vi "MTS_SaveImagePng.vi"(5 "Save .png":bool=TRUE, 6 "Tree Refnum":refnum<vi>, 7 ".pt3 File Name":path, 8 "error in":errorcluster, 11 "Image":i32[][](array[numeric])) -> (0 "error out":errorcluster)   [LabVIEW 8.6]
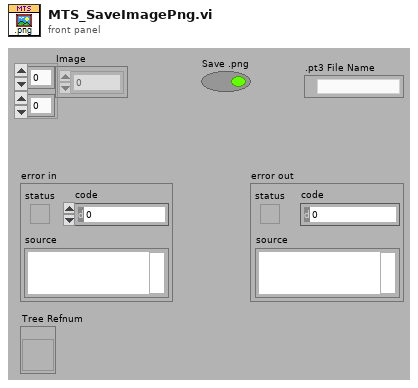
[diagram p1: front panel]
types:
  T1 = enum16{"unknown", "pt3 File", "png Image", "bmp Image"}
  T2 = enum16{"not a pt3 File", "Image File", "Point Measurement", "Auto Point"}
  T3 = typedef "Image Type" = u32
  T4 = typedef "IMAQ Image.ctl" = refnum<image>
  T5 = cluster{"File No":i32, "File Path":path, "Parent File":i32, "File Type":enum16{"unknown", "pt3 File", "png Image", "bmp Image"}, "Measurement Type":enum16{"not a pt3 File", "Image File", "Point Measurement", "Auto Point"}, "Upper Left":cluster{"x-Position":dbl, "y-Position":dbl, "z-Position":dbl}, "Pixels":i32[], "Picture Size":dbl[], "Scan Axis":enum32{"x-y", "x-z", "y-z"}}
  T6 = cluster{"x-Position":dbl, "y-Position":dbl, "z-Position":dbl}
  T7 = cluster{"Picture Size":dbl[], "Pixels":i32[], "Upper Left":cluster{"x-Position":dbl, "y-Position":dbl, "z-Position":dbl}}
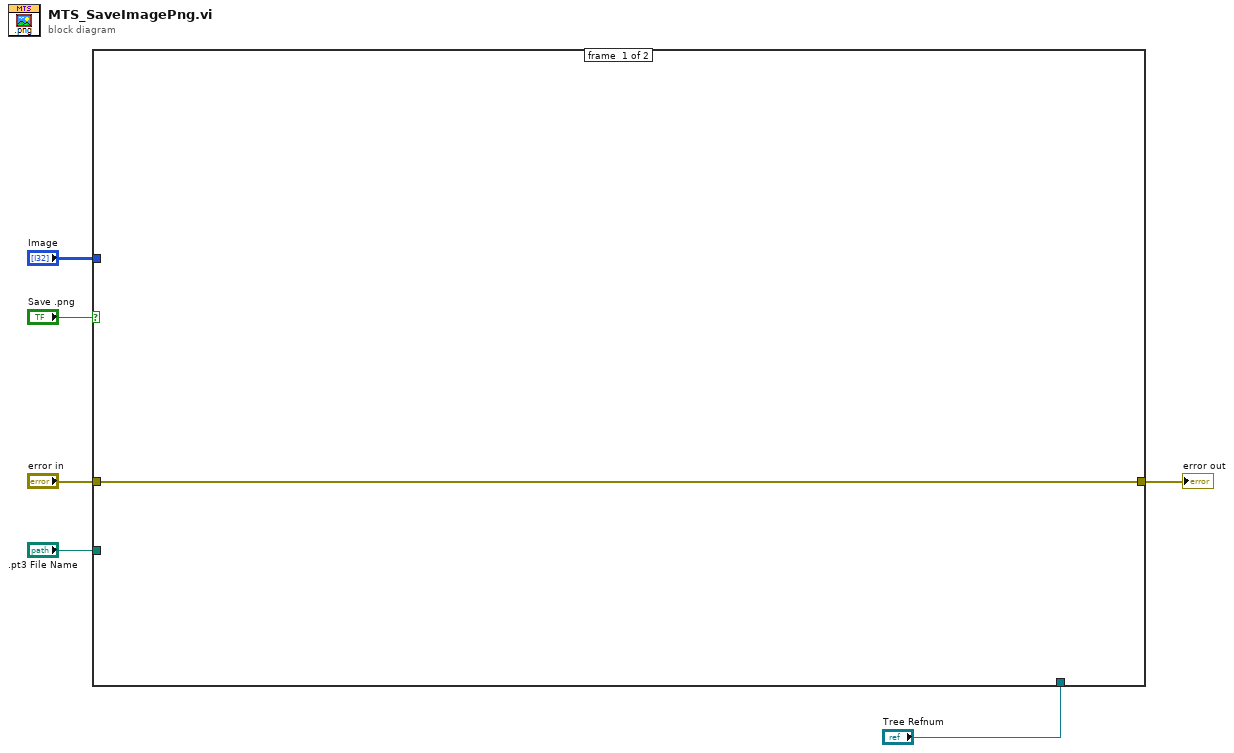
[diagram p0: block diagram]
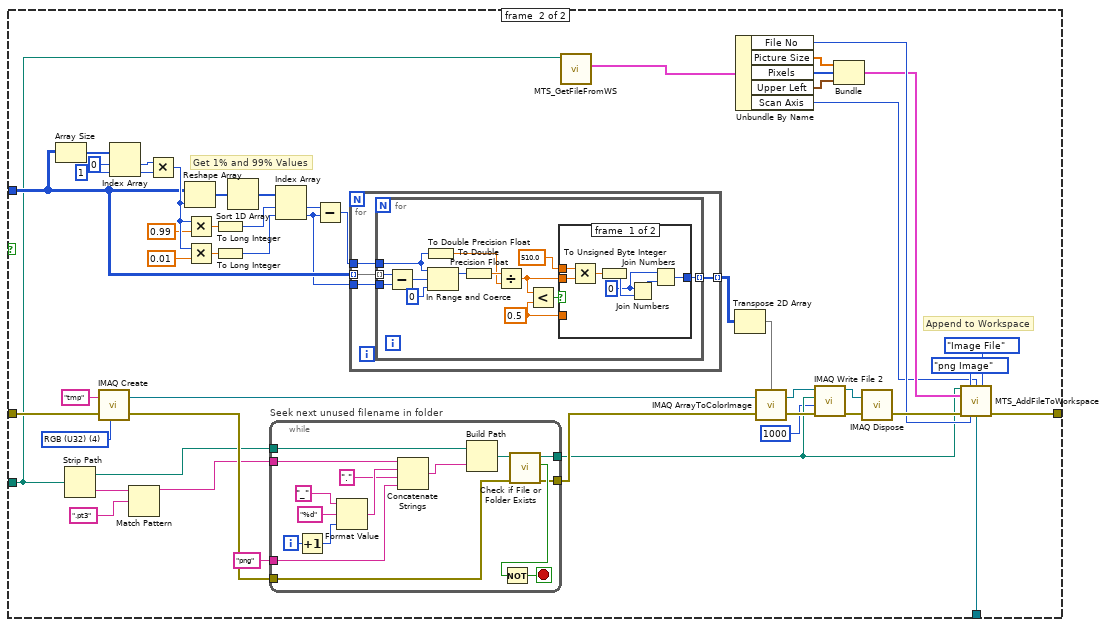
[diagram p2: hidden frame]
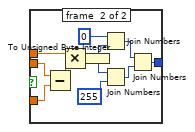
[diagram p3: hidden frame]
diagram:
  n1 = case shown="True" "Save .png" {
    tunnel: "Image" -> [_ w40]
    tunnel: "error in" -> [w7 w43]
    tunnel: [w7 w23] -> w3
    tunnel: ".pt3 File Name" -> [_ w9]
    tunnel: "Tree Refnum" -> [_ w22]
    frame #0 {
    }
    frame #1 {
      w41 = T3 4 items=["Grayscale (U8)", "Grayscale (I16)", "Grayscale (SGL)", "Complex (CSG)", "RGB (U32)", "HSL (U32)", "RGB (U64)", "Grayscale (U16)"] ("Image Type")
      # "Append to Workspace"
      # "Get 1% and 99% Values"
      n2 = Array Size(array=w40) -> (size(s)=w57:i32[])
      n3 = Strip Path(path=w9) -> (stripped path=w27:path, name=w31:string)
      n4 = call "IMAQ Create"("Image Name"="tmp", "Image Type"=w41, "error in (no error)"=w43) -> ("New Image"=w36:T4, "error out"=w29:errorcluster)  [unwired: 2 in]
      n5 = Index Array(array=w57, index #1=0 ("index"), index #2=1 ("index")) -> (element #1=w54:i32, element #2=w53:i32)
      n6 = Match Pattern(string=w31, regular expression=".pt3") -> (before substring=w26:string)  [unwired: 1 in, 3 out]
      n7 = Multiply(x=w54, y=w53) -> (x*y=w50:i32)
      n8 = Reshape Array(w40, w50) -> (w52:i32[])
      n9 = Multiply(x=w50, y=0.99) -> (x*y=w47:dbl)
      n10 = Multiply(x=w50, y=0.01) -> (x*y=w46:dbl)
      n11 = To Long Integer(number=w47) -> (32bit integer=w44:i32)
      n12 = To Long Integer(number=w46) -> (32bit integer=w45:i32)
      n13 = Sort 1D Array(array=w52) -> (sorted array=w51:i32[])
      n14 = while "Seek next unused filename in folder" {
        tunnel: w27 -> [w73]
        tunnel: [w68] -> w15
        tunnel: w29 -> [w67]
        tunnel: [w66] -> w28
        tunnel: w26 -> [w61]
        tunnel: "png" ("File Type") -> [w58]
        i -> [w63]
        stop <- w70 stop-if-true
        n15 = Increment(x=w63) -> (x+1=w62:i32)
        n16 = Format Value(string ("")="_", format string="%d", value (0)=w62) -> (output string=w64:string)
        n17 = Concatenate Strings(w61, w64, "." ("string"), w58) -> (w72:string)
        n18 = Build Path(base path=w73, name or relative path=w72) -> (appended path=w71:path)
        n19 = call <vilib>:"Check if File or Folder Exists.vi"("error in (no error)"=w67, "path"=w71) -> ("error out"=w66:errorcluster, "file or folder exists?"=w69:bool, "dup path"=w68:path)  [unwired: 7 in]
        n20 = Not(x=w69) -> (.not. x?=w70:bool)
      }
      n21 = Index Array(array=w51, index #1=w44, index #2=w45) -> (element #1=w39:i32, element #2=w38:i32)
      n22 = Subtract(x=w39, y=w38) -> (x-y=w37:i32)
      n23 = for {
        tunnel: w40 -> [w77] mode=indexing
        tunnel: w38 -> [w76]
        tunnel: w37 -> [w75]
        tunnel: [w74] -> w14 mode=indexing
        n24 = for {
          tunnel: w77 -> [w90] mode=indexing
          tunnel: w76 -> [w89]
          tunnel: w75 -> [w85]
          tunnel: [w79] -> w74 mode=indexing
          w78 = 0.5 ("y")
          n25 = Subtract(x=w90, y=w89) -> (x-y=w88:i32)
          n26 = To Double Precision Float(number=w85) -> (double precision float=w83:dbl)
          n27 = In Range and Coerce(upper limit=w85, x=w88, lower limit=0) -> (coerced(x)=w86:i32)  [unwired: 1 out]
          n28 = To Double Precision Float(number=w86) -> (double precision float=w84:dbl)
          n29 = Divide(x=w84, y=w83) -> (x/y=w81:dbl)
          n30 = Less?(x=w81, y=w78) -> (x < y?=w82:bool)
          n31 = case shown="False" w82 {
            tunnel: w81 -> [w97 w104]
            tunnel: 510.0 ("y") -> [w96 w108]
            tunnel: [w92 w105] -> w79
            tunnel: w78 -> [_ w103]
            frame #0 {
              w91 = u8 0 ("hi")
              n32 = Multiply(x=w96, y=w97) -> (x*y=w95:dbl)
              n33 = To Unsigned Byte Integer(number=w95) -> (unsigned 8bit integer=w93:u8)
              n34 = Join Numbers(hi=w91, lo=w93) -> ((hi.lo)=w94:u16)
              n35 = Join Numbers(hi=w91, lo=w94) -> ((hi.lo)=w92:u32)
            }
            frame #1 {
              n36 = Subtract(x=w104, y=w103) -> (x-y=w102:dbl)
              n37 = Multiply(x=w108, y=w102) -> (x*y=w107:dbl)
              n38 = To Unsigned Byte Integer(number=w107) -> (unsigned 8bit integer=w101:u8)
              n39 = Join Numbers(hi=u8 0, lo=w101) -> ((hi.lo)=w100:u16)
              n40 = Join Numbers(hi=w101, lo=u8 255) -> ((hi.lo)=w106:u16)
              n41 = Join Numbers(hi=w100, lo=w106) -> ((hi.lo)=w105:u32)
            }
          }
        }
      }
      n42 = call "MTS_GetFileFromWS.vi"(".pt3 File Name"=w9) -> ("File Header"=w10:T5)  [unwired: 9 in, 1 out]
      n43 = Transpose 2D Array(2D array=w14) -> (transposed array=w13:u32[][])
      n44 = Unbundle By Name(w10) -> ("File No"=w17:i32, "Picture Size"=w20:dbl[], "Pixels"=w19:i32[], "Upper Left"=w18:T6, "Scan Axis"=w8:enum32{"x-y", "x-z", "y-z"})
      n45 = call "IMAQ ArrayToColorImage"("Image Pixels (U32)"=w13, "Image"=w36, "error in (no error)"=w28) -> ("Image Out"=w33:T4, "error out"=w35:errorcluster)  [unwired: 2 in]
      n46 = call-poly "IMAQ Write File 2"("error in (no error)"=w35, "Image Quality"=u32 1000, "File Path"=w15, "Image"=w33) -> ("error out"=w34:errorcluster, "Image Out (duplicate)"=w32:T4)  [unwired: 6 in]
      n47 = Bundle("Picture Size"=w20, "Pixels"=w19, "Upper Left"=w18) -> (w16:T7)  [unwired: 1 in]
      n48 = call "IMAQ Dispose"("Image"=w32, "error in (no error)"=w34) -> ("error out"=w24:errorcluster)  [unwired: 4 in]
      n49 = call "MTS_AddFileToWorkspace.vi"("File Name"=w15, "File Type"=T1."png Image", "Scan Axis"=w8, "Measurement Type"=T2."Image File", "File Info"=w16, "error in (no error)"=w24, "Parent"=w17, "Tree Refnum"=w22) -> ("error out"=w23:errorcluster)  [unwired: 5 in, 2 out]
    }
  }
  "error out" <- w3
